vi "Check Local Files.vi"(8 "error in (no error)":errorcluster, 11 "Sequencing Control in":refnum<class "Sequencing Control.lvclass">) -> (0 "error out":errorcluster, 3 "Sequencing Control out":refnum<class "Sequencing Control.lvclass">)   [LabVIEW 2023, in "VolatusSeqGUI.lvlib" / "Sequencing Control.lvclass"]
uses:
  Sequencing Control.lvclass
  Sequencing Control.lvclass/Sequencing Control.ctl
  <vilib>/Utility/miscctls.llb/LVMapReplaceAction.ctl
  VolatusSeqConfig/Sequence Config/Sequence Config.lvclass
  VolatusSeqConfig/Sequence Validation/Sequence Validation.lvclass
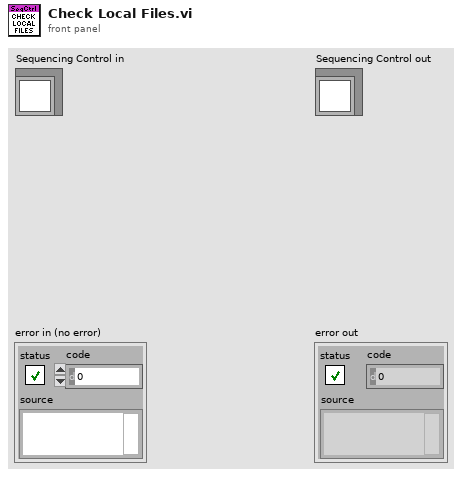
[diagram p1: front panel]
types:
  T1 = typedef "VolatusSeqGUI.lvlib/Sequencing Control.lvclass/Local File Info.ctl" = cluster{"Path":path, "Name":string, "CRC":u32, "Last Modified":timestamp, "error":errorcluster}
  T2 = typedef "LVMapReplaceAction.ctl" = enum32{"Modify Entry only if found", "Add or Modify Entry", "Delete Entry"}
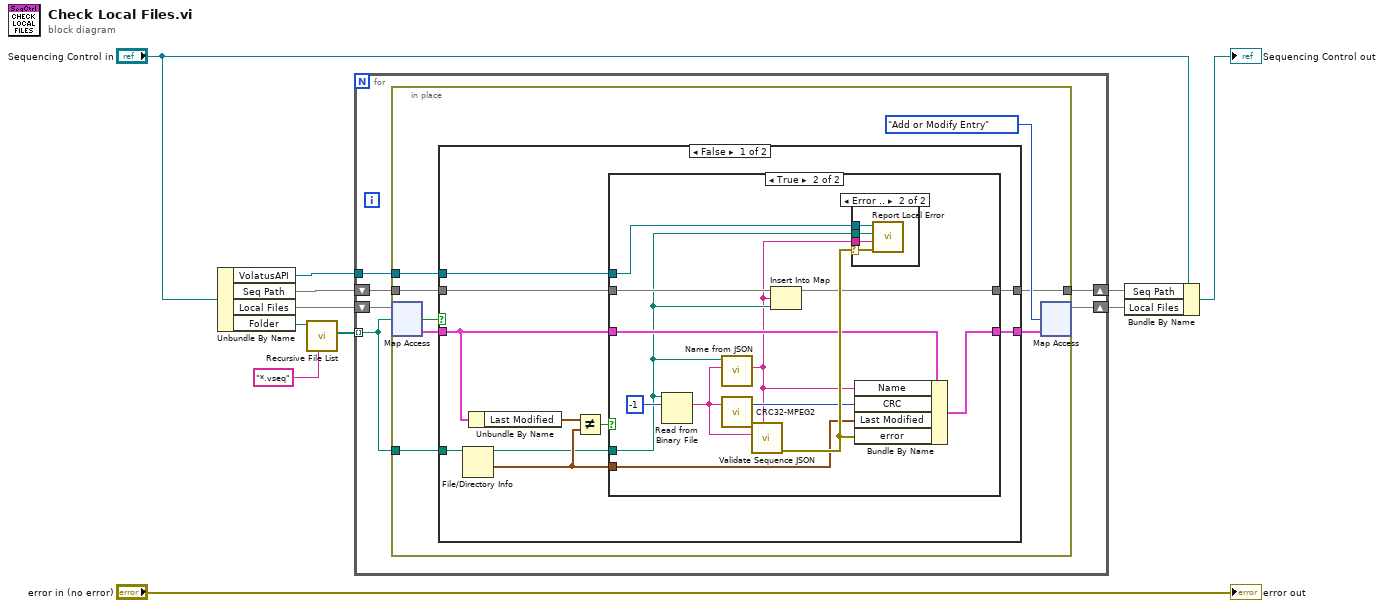
[diagram p0: block diagram]
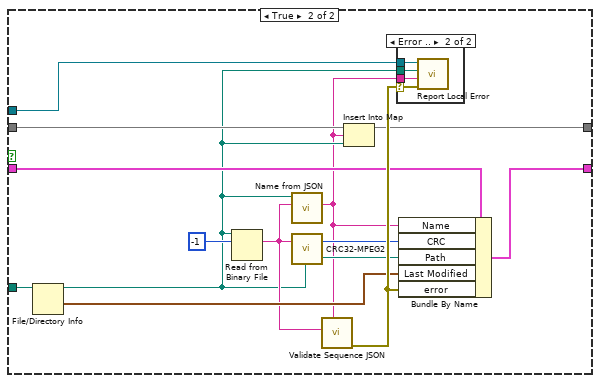
[diagram p4: hidden frame]
diagram:
  n1 = Unbundle By Name("Sequencing Control in") -> ("VolatusAPI"=w1:refnum<class "VolatusAPI.lvclass">, "Seq Path"=w3:map{string, path}, "Local Files"=w7:map{path, T1}, "Folder"=w10:path)
  n2 = call <vilib>:"Recursive File List.vi"("pattern"="*.vseq", "Folder Path"=w10) -> ("All Files in Dir"=w8:path[])  [unwired: 5 in, 4 out]
  n3 = for {
    tunnel: w8 -> [w16] mode=indexing
    shift-right: [w15] -> w6
    shift-left: w7 -> [w17]
    shift-right: [w13] -> w2
    shift-left: w3 -> [w14]
    tunnel: w1 -> [w12]
    n4 = in-place {
      in-place-border: w16 -> [w22]
      in-place-border: w14 -> [w20]
      in-place-border: [w19] -> w13
      in-place-border: w12 -> [w18]
      n5 = in-place-map #1(w17, w16) -> (w24:T1, w23:bool)  [unwired: 1 in]
      n6 = case shown="False" w23 {
        tunnel: w24 -> [w31 w63]
        tunnel: w22 -> [w35 w62]
        tunnel: [w29 w60] -> w21
        tunnel: w20 -> [w28 w59]
        tunnel: [w27 w58] -> w19
        tunnel: w18 -> [w26 w56]
        frame False {
          n7 = File/Directory Info(path=w35) -> (path out=w30:path, last mod=w32:timestamp)  [unwired: 1 in, 5 out]
          n8 = Unbundle By Name(w31) -> ("Last Modified"=w34:timestamp)
          n9 = Not Equal?(x=w34, y=w32) -> (x != y?=w33:bool)
          n10 = case shown="True" w33 {
            tunnel: w32 -> [_ w45]
            tunnel: w31 -> [w37 w47]
            tunnel: w30 -> [_ w39]
            tunnel: [w37 w44] -> w29
            tunnel: w28 -> [w36 w43]
            tunnel: [w36 w42] -> w27
            tunnel: w26 -> [_ w40]
            frame False {
            }
            frame True {
              n11 = Read from Binary File(10:-1 ("count (1)"), 11:w39) -> (2:w41:string)  [unwired: 4 in, 3 out]
              n12 = call "Name from JSON.vi"("JSON"=w41, "Path"=w39) -> ("Name"=w38:string)  [unwired: 8 in, 1 out]
              n13 = call "CRC32-MPEG2.vi"("Data In"=w41) -> ("CRC"=w46:u32)  [unwired: 6 in]
              n14 = call "Validate Sequence JSON.vi"("Fallback Name"=w38, "JSON"=w41) -> ("error out"=w49:errorcluster)  [unwired: 9 in]
              n15 = Insert Into Map(map in=w43, key=w38, value=w39) -> (map out=w42:map{string, path})  [unwired: 2 out]
              n16 = case shown="Error .." w49 {
                selector: w49 -> [_ w50]
                tunnel: w38 -> [_ w53]
                tunnel: w39 -> [_ w52]
                tunnel: w40 -> [_ w51]
                frame No Error {
                }
                frame Error {
                  n17 = call "Report Local Error.vi"("error in (no error)"=w50, "Name"=w53, "Path"=w52, "VolatusAPI"=w51) -> ()  [unwired: 8 in]
                }
              }
              n18 = Bundle By Name(cluster=w47, "Name"=w38, "CRC"=w46, "Last Modified"=w45, "error"=w49) -> (w44:T1)
            }
          }
        }
        frame True {
          n19 = File/Directory Info(path=w62) -> (path out=w55:path, last mod=w61:timestamp)  [unwired: 1 in, 5 out]
          n20 = Read from Binary File(10:-1 ("count (1)"), 11:w55) -> (2:w57:string)  [unwired: 4 in, 3 out]
          n21 = call "Name from JSON.vi"("JSON"=w57, "Path"=w55) -> ("Name"=w54:string)  [unwired: 8 in, 1 out]
          n22 = call "CRC32-MPEG2.vi"("Data In"=w57) -> ("CRC"=w64:u32)  [unwired: 6 in]
          n23 = call "Validate Sequence JSON.vi"("Fallback Name"=w54, "JSON"=w57) -> ("error out"=w66:errorcluster)  [unwired: 9 in]
          n24 = Insert Into Map(map in=w59, key=w54, value=w55) -> (map out=w58:map{string, path})  [unwired: 2 out]
          n25 = case shown="Error .." w66 {
            selector: w66 -> [_ w67]
            tunnel: w54 -> [_ w70]
            tunnel: w55 -> [_ w69]
            tunnel: w56 -> [_ w68]
            frame No Error {
            }
            frame Error {
              n26 = call "Report Local Error.vi"("error in (no error)"=w67, "Name"=w70, "Path"=w69, "VolatusAPI"=w68) -> ()  [unwired: 8 in]
            }
          }
          n27 = Bundle By Name(cluster=w63, "Name"=w54, "CRC"=w64, "Path"=w55, "Last Modified"=w61, "error"=w66) -> (w60:T1)
        }
      }
      n28 = in-place-map #1(w21, LVMapReplaceAction."Add or Modify Entry" ("action")) -> (w15:map{path, T1})  [unwired: 2 out]
    }
  }
  n29 = Bundle By Name(cluster="Sequencing Control in", "Seq Path"=w2, "Local Files"=w6) -> (→"Sequencing Control out":refnum<class "Sequencing Control.lvclass">)
  "error out" <- "error in (no error)"
